vi "AutoMechs.vi"(6 "Wrist":dbl format="%#_13g", 7 "Time":u32=1000, 8 "WristMode":bool, 9 "Intake":dbl format="%#_13g", 10 "Lift":dbl format="%#_13g", 11 "LiftMode":bool) -> ()   [LabVIEW 2017]
uses:
  Phoenix-LabVIEW/Motor Controller/Controls/CTRE_Phoenix_MotorControl_ControlMode.ctl
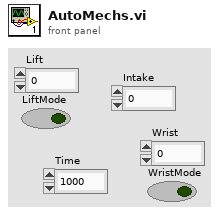
[diagram p1: front panel]
types:
  T1 = typedef "CTRE_Phoenix_MotorControl_ControlMode.ctl" = u16
  T2 = typedef "WPI_MotorControlDeviceRef.ctl" = cluster{"DeviceStatus":errorcluster, "Type":T3, "PWM":cluster{"PWM Channel":T4, "DeadBand":T5}, "CAN":cluster{"Device Number":u8, "SetOutput VI Ref":variant, "GetOutput VI Ref":variant, "Enable VI Ref":variant, "Disable VI Ref":variant, "Data":variant}, "Invert":bool, "DIO PWM":cluster{"PWM \"Enable\" Channel":T4, "DIOChannel":T6, "PWM Rate":dbl}}
  T3 = typedef "WPI_MotorControlType.ctl" = enum16{"PWM", "CAN", "DIO PWM"}
  T4 = typedef "FPGA_DIOPWMChannel.ctl" = enum8{"PWM 0", "PWM 1", "PWM 2", "PWM 3", "PWM 4", "PWM 5", "PWM 6", "PWM 7", "PWM 8", "PWM 9", "PWM MXP 0", "PWM MXP 1", "PWM MXP 2", "PWM MXP 3", "PWM MXP 4", "PWM MXP 5", "PWM MXP 6", "PWM MXP 7", "PWM MXP 8", "PWM MXP 9", "Invalid"}
  T5 = typedef "WPI_PWMDeadband.ctl" = cluster{"Name":string, "maxPositivePwm":i32, "minPositivePwm":i32, "centerPwm":i32, "maxNegativePwm":i32, "minNegativePwm":i32, "angularRange":u16}
  T6 = typedef "FPGA_DIOChannel.ctl" = enum8{"DIO 0", "DIO 1", "DIO 2", "DIO 3", "DIO 4", "DIO 5", "DIO 6", "DIO 7", "DIO 8", "DIO 9", "DIO MXP 0", "DIO MXP 1", "DIO MXP 2", "DIO MXP 3", "DIO MXP 4", "DIO MXP 5", "DIO MXP 6", "DIO MXP 7", "DIO MXP 8", "DIO MXP 9", "DIO MXP 10", "DIO MXP 11", "DIO MXP 12", "DIO MXP 13", "DIO MXP 14", "DIO MXP 15", "SPI Port CS1", "SPI Port CS2", "SPI Port CS3", "SPI Port MISO", "SPI Port MOSI", "Invalid"}
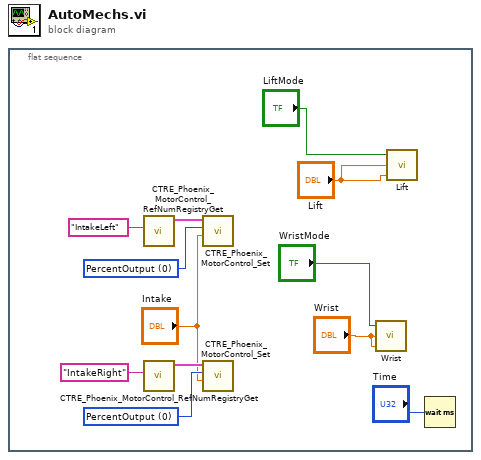
[diagram p0: block diagram]
diagram:
  n1 = flat-sequence {
    frame #0 {
      w7 = T1 0 items=["PercentOutput"=0, "Position"=1, "Velocity"=2, "Current"=3, "Follower"=5, "MotionProfile"=6, "MotionMagic"=7, "MotionMagicArc"=8, "MotionProfileArc"=10, "Disabled"=15] ("Control Mode")
      w10 = T1 0 items=["PercentOutput"=0, "Position"=1, "Velocity"=2, "Current"=3, "Follower"=5, "MotionProfile"=6, "MotionMagic"=7, "MotionMagicArc"=8, "MotionProfileArc"=10, "Disabled"=15] ("Control Mode")
      n2 = call "CTRE_Phoenix_MotorControl_RefNumRegistryGet.vi"("refnum name"="IntakeLeft") -> ("PhoenixMotorControlDevRef"=w12:T2)  [unwired: 9 in, 1 out]
      n3 = call "CTRE_Phoenix_MotorControl_RefNumRegistryGet.vi"("refnum name"="IntakeRight") -> ("PhoenixMotorControlDevRef"=w9:T2)  [unwired: 9 in, 1 out]
      n4 = call "CTRE_Phoenix_MotorControl_Set.vi"("Output"="Intake", "Control Mode"=w10, "PhoenixMotorControlDevRef"=w12) -> ()  [unwired: 7 in, 2 out]
      n5 = call "CTRE_Phoenix_MotorControl_Set.vi"("Output"="Intake", "Control Mode"=w7, "PhoenixMotorControlDevRef"=w9) -> ()  [unwired: 7 in, 2 out]
      n6 = call "Wrist.vi"("WristInput"="Wrist", "WristSetpoint"="Wrist", "WristSweet"="WristMode") -> ()
      n7 = call "Lift.vi"("LiftInput"="Lift", "LiftSet"="Lift", "LiftSweet"="LiftMode") -> ()
      n8 = Wait (ms)(milliseconds to wait="Time") -> ()  [unwired: 1 out]
    }
  }
